vi "Filter Data.vi"(8 "error in (no error)":errorcluster, 10 "Debug Data In":refnum<class "Debug Data.lvclass">[](array[class]), 11 "Filter in":refnum<class "Filter.lvclass">) -> (0 "error out":errorcluster, 2 "Debug Data Out":refnum<class "Debug Data.lvclass">[](array[class]), 3 "Filter out":refnum<class "Filter.lvclass">)   [LabVIEW 2020, in "Filter.lvclass"]
uses:
  Filter.lvclass
  Debug Data/Debug Data.lvclass
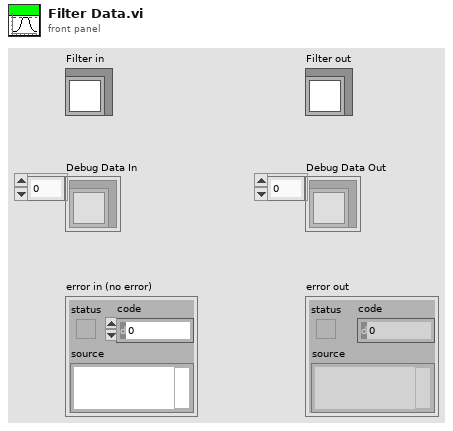
[diagram p1: front panel]
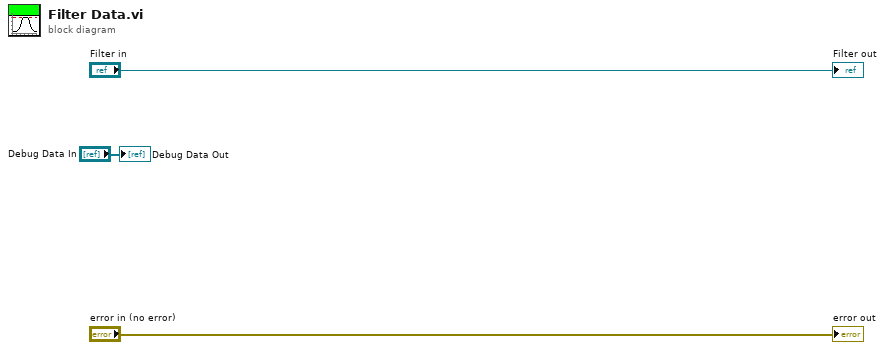
[diagram p0: block diagram]
diagram:
  "error out" <- "error in (no error)"
  "Filter out" <- "Filter in"
  "Debug Data Out" <- "Debug Data In"
